vi "MotorSpeedv2.vi"(6 "MotrSpdInfo":T1={"TrgtCounts"=0, "Accel?"=FALSE, "CurrCounts"=0.0, "SlowRng"=572.75, "MinPwr"=572.75} {"MinPwr" format="%#_13g"; "SlowRng" format="%#_13g"}, 8 "RightSpdIn":dbl, 11 "LeftSpdIn":dbl) -> (0 "RightSpdOut":dbl, 3 "LeftSpdOut":dbl)   [LabVIEW 2017]
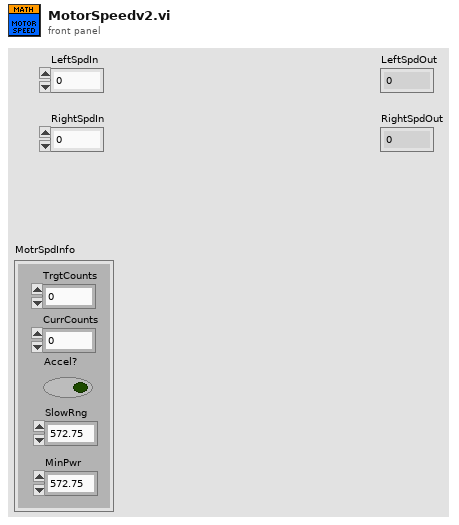
[diagram p1: front panel]
types:
  T1 = cluster{"TrgtCounts":i32, "Accel?":bool, "CurrCounts":dbl, "SlowRng":dbl, "MinPwr":dbl}
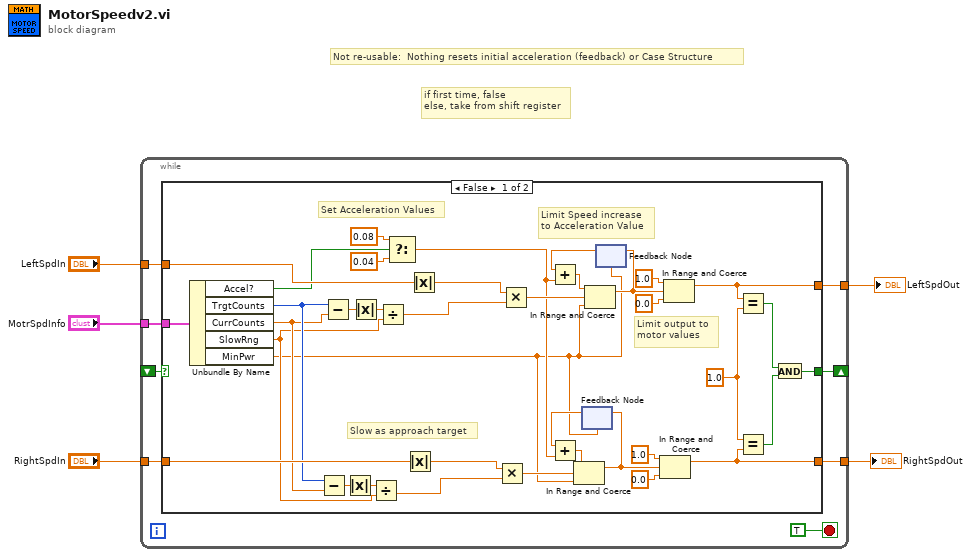
[diagram p0: block diagram]
diagram:
  # "if first time, false\nelse, take from shift register"
  # "Not re-usable:  Nothing resets initial acceleration (feedback) or Case Structure"
  n1 = while {
    tunnel: [w13] -> w5
    tunnel: "LeftSpdIn" -> [w12]
    tunnel: "RightSpdIn" -> [w11]
    tunnel: [w10] -> w2
    tunnel: "MotrSpdInfo" -> [w9]
    shift-right: [w8] -> _
    shift-left: _ -> [w7]
    stop <- TRUE stop-if-true
    n2 = case shown="False" w7 {
      selector: w7 -> [_ w53]
      tunnel: [w18 w51] -> w13
      tunnel: w12 -> [w39 w51]
      tunnel: w11 -> [w38 w52]
      tunnel: [w19 w52] -> w10
      tunnel: w9 -> [w28 _]
      tunnel: [w14 w53] -> w8
      frame False {
        w17 = 1.0 ("upper limit")
        # "Limit output to\nmotor values"
        # "Limit Speed increase\nto Acceleration Value"
        # "Slow as approach target"
        # "Set Acceleration Values"
        n3 = Unbundle By Name(w28) -> ("Accel?"=w24:bool, "TrgtCounts"=w27:i32, "CurrCounts"=w26:dbl, "SlowRng"=w25:dbl, "MinPwr"=w22:dbl)
        n4 = Subtract(x=w27, y=w26) -> (x-y=w30:dbl)
        n5 = Subtract(x=w27, y=w26) -> (x-y=w47:dbl)
        n6 = Absolute Value(x=w30) -> (abs(x)=w31:dbl)
        n7 = Absolute Value(x=w47) -> (abs(x)=w46:dbl)
        n8 = Divide(x=w31, y=w25) -> (x/y=w20:dbl)
        n9 = Divide(x=w46, y=w25) -> (x/y=w21:dbl)
        n10 = Select(t=0.08, s=w24, f=0.04) -> (s? t:f=w23:dbl)
        n11 = Absolute Value(x=w38) -> (abs(x)=w29:dbl)
        n12 = Absolute Value(x=w39) -> (abs(x)=w48:dbl)
        n13 = Multiply(x=w29, y=w20) -> (x*y=w34:dbl)
        n14 = Multiply(x=w48, y=w21) -> (x*y=w43:dbl)
        n15 = feedback #1(w22) -> (w33:dbl)
        n16 = Add(x=w33, y=w23) -> (x+y=w32:dbl)
        n17 = In Range and Coerce(upper limit=w32, x=w34, lower limit=w22) -> (coerced(x)=w37:dbl)  [unwired: 1 out]
        n18 = feedback-in #1(w37) -> ()
        n19 = feedback #2(w22) -> (w44:dbl)
        n20 = Add(x=w44, y=w23) -> (x+y=w45:dbl)
        n21 = In Range and Coerce(upper limit=w45, x=w43, lower limit=w22) -> (coerced(x)=w40:dbl)  [unwired: 1 out]
        n22 = feedback-in #2(w40) -> ()
        n23 = In Range and Coerce(upper limit=1.0, x=w37, lower limit=0.0) -> (coerced(x)=w19:dbl)  [unwired: 1 out]
        n24 = In Range and Coerce(upper limit=1.0, x=w40, lower limit=0.0) -> (coerced(x)=w18:dbl)  [unwired: 1 out]
        n25 = Equal?(x=w18, y=w17) -> (x = y?=w16:bool)
        n26 = Equal?(x=w17, y=w19) -> (x = y?=w15:bool)
        n27 = And(x=w16, y=w15) -> (x .and. y?=w14:bool)
      }
      frame True {
      }
    }
  }
  "LeftSpdOut" <- w5
  "RightSpdOut" <- w2
